vi "Configure test.vi"(6 "Assert VI Path":path, 7 "Existing Queue Elements":string, 8 "error in (no error)":errorcluster, 11 "Basic Str Equal in":refnum<class "Str Equal.lvclass">) -> (0 "error out":errorcluster, 3 "Basic Str Equal out":refnum<class "Str Equal.lvclass">)   [LabVIEW 2018, in "Str Equal.lvclass"]
uses:
  Str Equal.lvclass
  fef8068f-c153-4770-8ede-b17d1752ce72.vi
  <vilib>/JDP Science/JSONtext/Find Item.vi
  fef8068f-c153-4770-8ede-b17d1752ce72.vi/b1ac4bf6-6559-47d3-a12b-3584baa2ec64.vi
  fef8068f-c153-4770-8ede-b17d1752ce72.vi/e17888c3-9d02-4c2c-a06f-7dfeb58e08f7.vi
  <vilib>/JDP Science/JSONtext/String Subset.vi
  Test Class String IDs.vi
  <vilib>/JDP Science/JSONtext/Parsing/Parse Full Path or Item Name.vi
  <vilib>/JDP Science/JSONtext/Offset/Find Item Locations by Path.vi
  <vilib>/JDP Science/JSONtext/JSON text to Variant.vi
  <vilib>/JDP Science/JSONtext/Variant to JSON Text.vi
  <vilib>/JDP Science/JSONtext/Set Item.vi
  String.lvclass
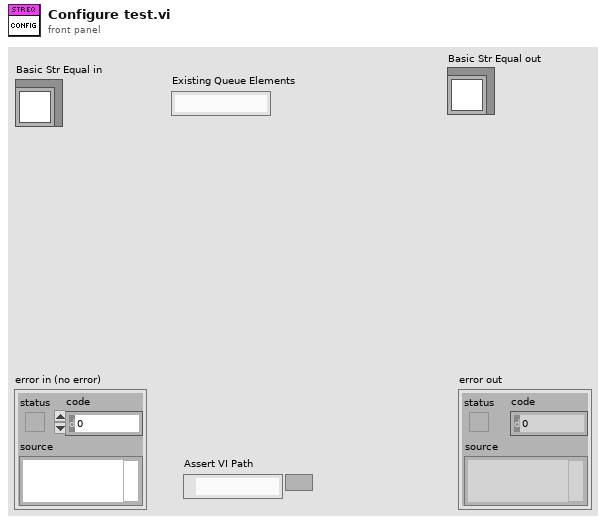
[diagram p1: front panel]
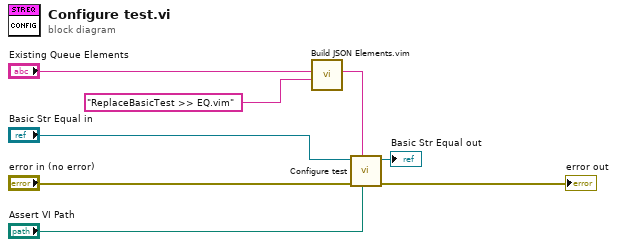
[diagram p0: block diagram]
diagram:
  n1 = call "Build JSON Elements.vim"("Append Element(s)"="ReplaceBasicTest >> EQ.vim", "JSON Elements in ({})"="Existing Queue Elements") -> ("JSON Elements out"=w2:string)  [unwired: 9 in]
  n2 = call-parent "Configure test.vi"("Assert VI Path"="Assert VI Path", "Existing Queue Elements"=w2, "error in (no error)"="error in (no error)", "Basic String in"="Basic Str Equal in") -> ("error out"=→"error out":errorcluster, "Basic String out"=→"Basic Str Equal out":refnum<class "Str Equal.lvclass">)  [unwired: 6 in]
